vi "Data Channel Page.vi"(8 "error in (no error)":errorcluster, 11 "Node Ptr":T2 format="%.0x") -> (0 "error out":errorcluster)   [LabVIEW 2021, in "DSF System Explorer.lvlib"]
uses:
  DSF System Explorer.lvlib
  <vilib>/NI VeriStand/Custom Device API/Custom Device Item Ref.ctl
  Includes/DSF Core.lvlibp/Classes/Component User Interface/UI Type.ctl
  <vilib>/NI VeriStand/Custom Device API/Custom Device API.lvlib
  Shared/DSF Shared.lvlib
  Includes/DSF Core.lvlibp/Classes/Component User Interface/Component User Interfaces.lvclass
  Includes/DSF Core.lvlibp/Classes/User Interface/User Interface.lvclass
panel:
  in  "Tab Control":enum32{"Settings"}(tab)
  in  "Default Value":dbl
  in  "Units":string
  out "Direction":enum16{"Tx", "Rx"}(ring)
  in  "Engine Data Type":T1(ring)
  in  "String Data Type":T1(ring)
  in  "String Offset":u64 format="%d bytes"
  in  "Header":cluster{"Section Name":string}={"Section Name"="Data Channel"}
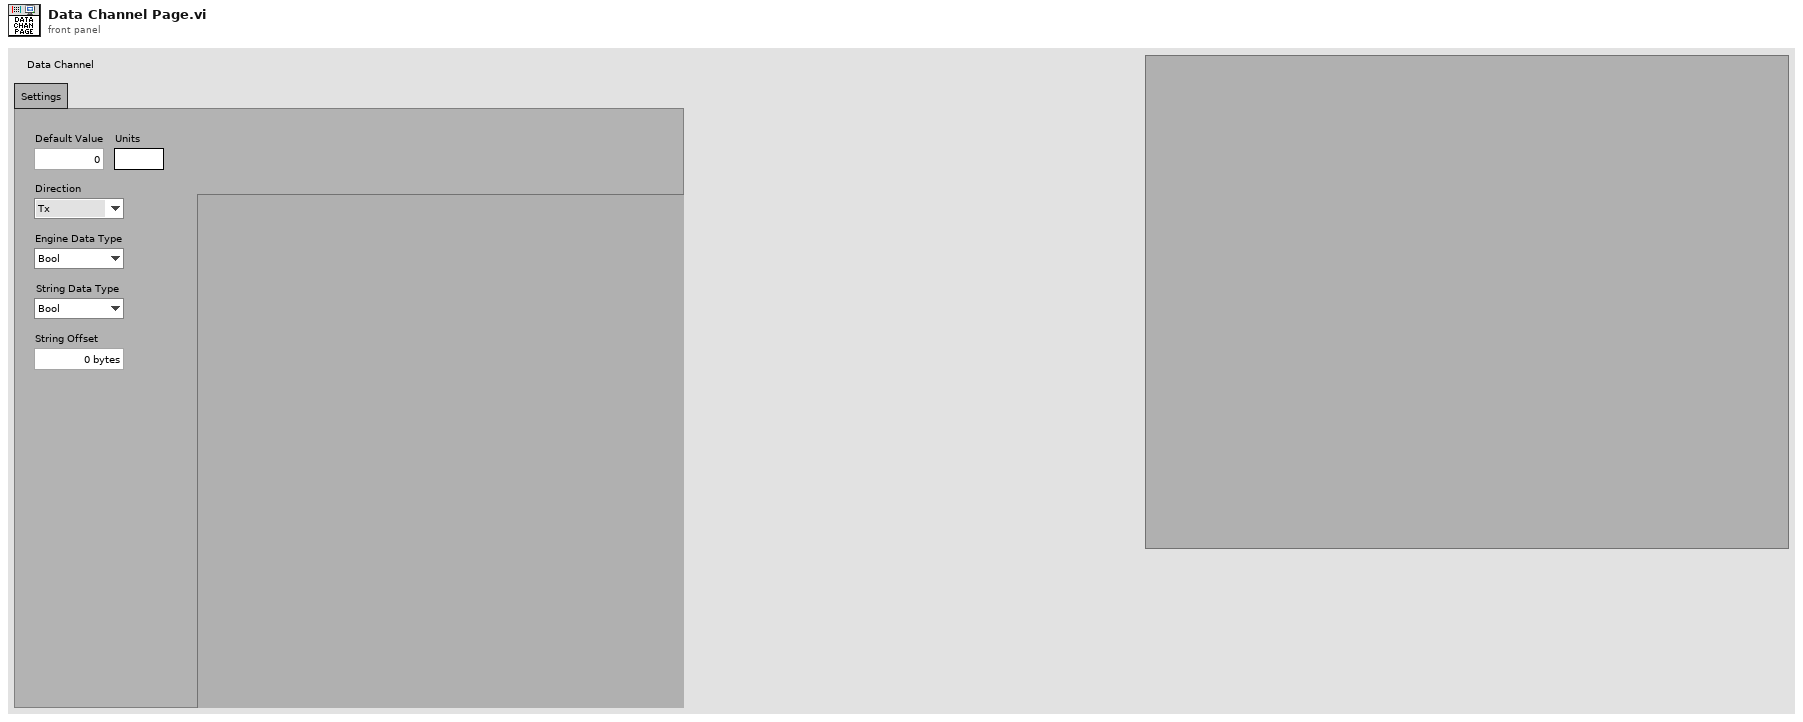
[diagram p1: front panel]
types:
  T1 = enum8{"Bool", "SGL", "DBL", "I8", "I16", "I32", "I64", "U8", "U16", "U32", "U64"}
  T2 = typedef "Custom Device API.lvlib/Custom Device Item Ref.ctl" = u64
  T3 = typedef "DSF Core.lvlibp/Component User Interfaces.lvclass/UI Type.ctl" = enum16{"Plugin", "Thread", "Rx Group", "Tx Group", "Rx Transfer", "Tx Transfer", "Rx Channel", "Tx Channel"}
  T4 = typedef "DSF Core.lvlibp/Channel Configuration.lvclass/Core Channel Configuration.ctl" = cluster{"name":string, "units":string, "engine data type":T5, "string data type":T5, "string offset":u64}
  T5 = typedef "DSF Core.lvlibp/DSF Data Type.ctl" = enum8{"Bool", "SGL", "DBL", "I8", "I16", "I32", "I64", "U8", "U16", "U32", "U64"}
  T6 = typedef "Custom Device API.lvlib/Custom Device Channel.ctl" = cluster{"Type":T7, "Units":string, "Default Value":dbl, "Faultable":bool, "Scalable":bool}
  T7 = typedef "Custom Device API.lvlib/Custom Device Channel Type.ctl" = enum16{"Input", "Output"}
  T8 = typedef "DSF Core.lvlibp/DSF Direction.ctl" = enum8{"Tx", "Rx"}
  T9 = typedef "DSF Core.lvlibp/User Interface Handler.lvclass/User Interface Ref.ctl" = refnum<vi>
  T10 = typedef "DSF Core.lvlibp/DSF Settings Info.ctl" = cluster{"component":string, "values":cluster{"key":string, "value":string}[]}
  T11 = typedef "Custom Device API.lvlib/Custom Device Commands.ctl" = enum16{"Default", "Item renamed", "Shutdown", "Dynamic button pressed"}
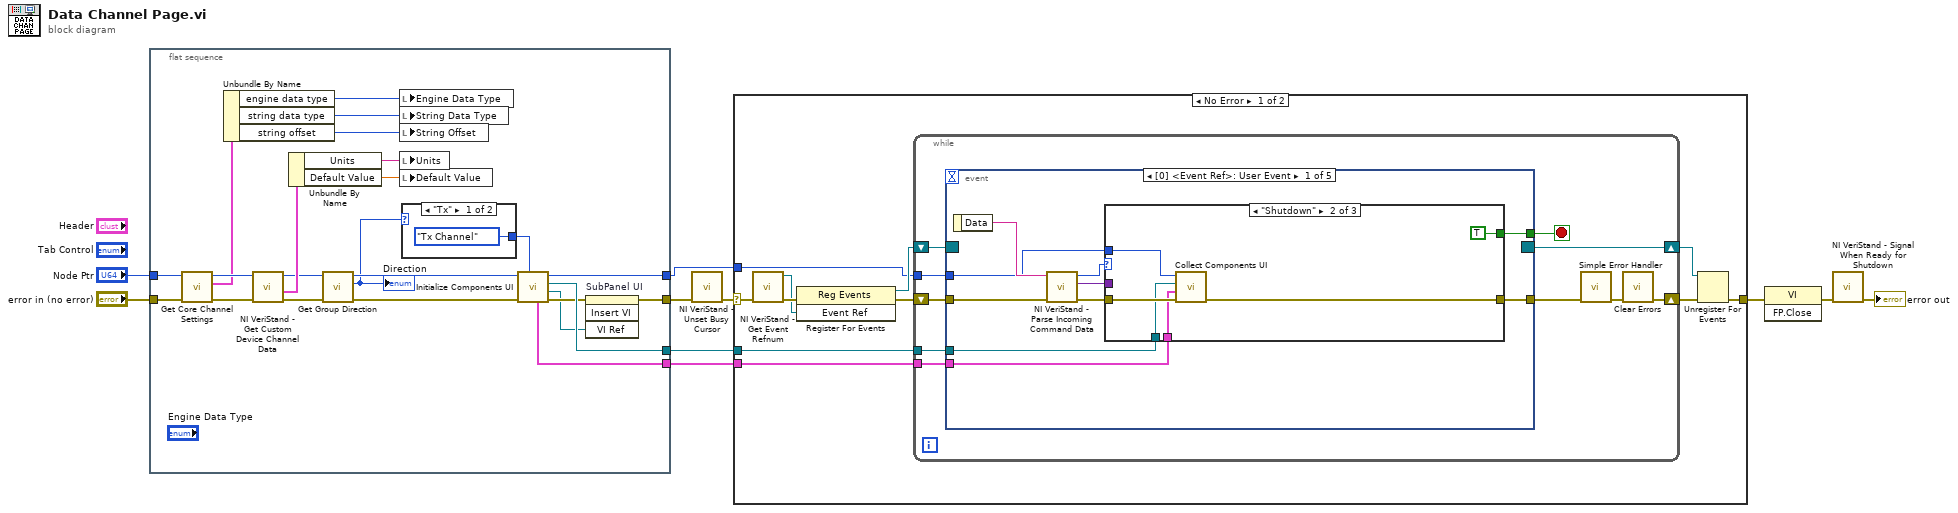
[diagram p0: block diagram]
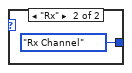
[diagram p2: hidden frame]
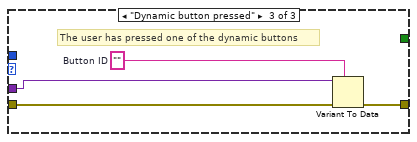
[diagram p4: hidden frame]
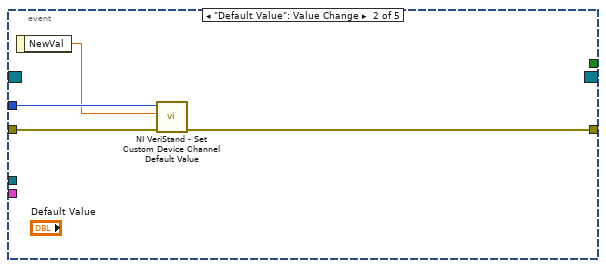
[diagram p5: hidden frame]
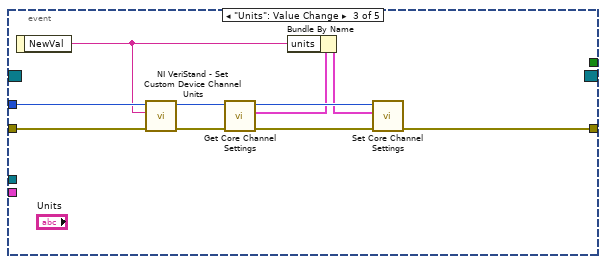
[diagram p6: hidden frame]
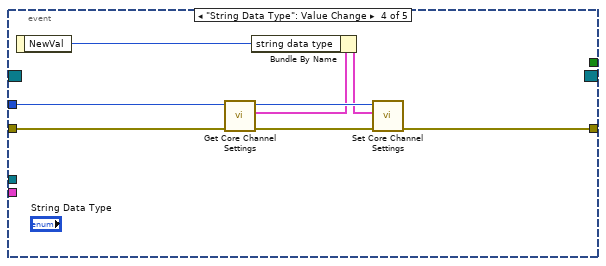
[diagram p7: hidden frame]
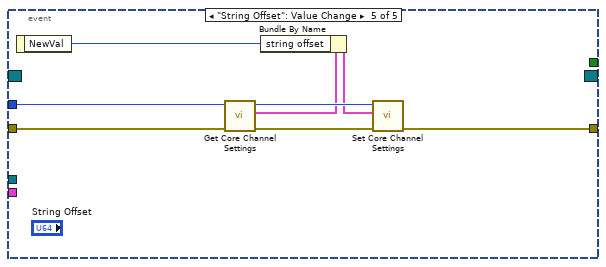
[diagram p8: hidden frame]
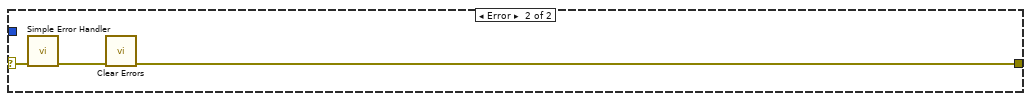
[diagram p9: hidden frame]
diagram:
  n1 = flat-sequence "Initialization code" {
    tunnel: "error in (no error)" -> [w31]
    tunnel: "Node Ptr" -> [w30]
    tunnel: [w12] -> w6
    tunnel: [w15] -> w3
    tunnel: [w16] -> w2
    tunnel: [w14] -> w1
    frame #0 {
      n2 = call "Get Core Channel Settings.vi"("error in (no error)"=w31, "Item Ref in"=w30) -> ("error out"=w29:errorcluster, "channel configuration"=w27:T4, "Item Ref out"=w28:T2)  [unwired: 7 in]
      n3 = Unbundle By Name(w27) -> ("engine data type"=w25:T5, "string data type"=w24:T5, "string offset"=w23:u64)
      n4 = call <vilib>:"NI VeriStand - Get Custom Device Channel Data.vi"("error in (no error)"=w29, "Channel Ref in"=w28) -> ("error out"=w22:errorcluster, "Channel"=w26:T6, "Channel Ref out"=w21:T2)  [unwired: 4 in, 3 out]
      n5 = Unbundle By Name(w26) -> ("Units"=w32:string, "Default Value"=w33:dbl)
      n6 = call "Get Group Direction.vi"("error in (no error)"=w22, "Item Ref in"=w21) -> ("error out"=w19:errorcluster, "direction"=w17:T8, "Item Ref out"=w18:T2)  [unwired: 6 in, 1 out]
      "Direction" <- w17
      n7 = local write "Engine Data Type"(w25) -> ()
      n8 = local write "String Data Type"(w24) -> ()
      n9 = local write "String Offset"(w23) -> ()
      n10 = local write "Units"(w32) -> ()
      n11 = local write "Default Value"(w33) -> ()
      n12 = case shown="\"Tx\"" w17 {
        tunnel: [UI_Type."Tx Channel" ("user interface type") UI_Type."Rx Channel" ("user interface type")] -> w20
        frame "Tx" {
        }
        frame "Rx" {
        }
      }
      n13 = call "Initialize Components UI.vi"("user interface type"=w20, "error in (no error)"=w19, "Item Ref in"=w18) -> ("error out"=w13:errorcluster, "active vi"=w11:T9, "User Interface Handler"=w16:refnum<class "User Interface Handler.lvclass">, "Item Ref out"=w15:T2, "component settings"=w14:T10[])  [unwired: 4 in]
      n14 = invoke on="SubPanel UI" class="SubPnl" method="Insert VI"(error in=w13, "VI Ref"=w11) -> (error out=w12:errorcluster)  [unwired: 2 in, 3 out]
    }
  }
  n15 = call <vilib>:"NI VeriStand - Unset Busy Cursor.vi"("error in (no error)"=w6) -> ("error out"=w5:errorcluster)  [unwired: 10 out]
  n16 = case shown="No Error" w5 {
    selector: w5 -> [w38 w110]
    tunnel: [w43 w108] -> w10
    tunnel: w3 -> [w39 _]
    tunnel: w2 -> [w37 _]
    tunnel: w1 -> [w36 _]
    frame No Error {
      n17 = call <vilib>:"NI VeriStand - Get Event Refnum.vi"("error in (no error)"=w38) -> ("error out"=w46:errorcluster, "Event Ref"=w42:refnum<user-event>)  [unwired: 9 out]
      n18 = register-events(error in=w46, w42) -> (reference out=w40:refnum<event-registration>, error out=w41:errorcluster)  [unwired: 1 in]
      n19 = while {
        tunnel: w39 -> [w52]
        shift-right: [w49] -> w44
        shift-left: w41 -> [w55]
        shift-right: [w56] -> w45
        shift-left: w40 -> [w54]
        tunnel: w37 -> [w48]
        tunnel: w36 -> [w47]
        stop <- w53 stop-if-true
        n20 = event shown="[0] <Event Ref>: User Event" {
          selector: w54 -> [_ _ _ _ _]
          dyn-events: [_ _ _ _ _] -> w56
          timeout: _ -> [_ _ _ _ _]
          tunnel: w55 -> [w66 w81 w91 w99 w107]
          tunnel: [w62 _ _ _ _] -> w53
          tunnel: [w61 w78 w82 w92 w100] -> w51
          tunnel: w52 -> [w60 w80 w90 w98 w106]
          tunnel: w48 -> [w58 _ _ _ _]
          tunnel: w47 -> [w57 _ _ _ _]
          event User Event {
            n21 = event-data() -> ("Data"=w65:string)  [unwired: 1 out]
            n22 = call <vilib>:"NI VeriStand - Parse Incoming Command Data.vi"("error in (no error)"=w66, "Incoming data"=w65) -> ("error out"=w64:errorcluster, "Outgoing data"=w59:variant, "Action"=w63:T11)  [unwired: 7 out]
            n23 = case shown="\"Shutdown\"" w63 {
              tunnel: w64 -> [w67 w72 w77]
              tunnel: [_ TRUE _] -> w62
              tunnel: [w67 w69 w74] -> w61
              tunnel: w60 -> [_ w71 _]
              tunnel: w59 -> [_ _ w76]
              tunnel: w58 -> [_ w70 _]
              tunnel: w57 -> [_ w68 _]
              frame "Default", Default {
              }
              frame "Shutdown" {
                n24 = call "Collect Components UI.vi"("error in (no error)"=w72, "current component settings"=w68, "User Interface Handler"=w70, "Item Ref in"=w71) -> ("error out"=w69:errorcluster)  [unwired: 6 in, 1 out]
              }
              frame "Dynamic button pressed" {
                w75 = ""  # Button ID
                # "The user has pressed one of the dynamic buttons"
                n25 = Variant To Data(error in=w77, type=w75, Variant=w76) -> (error out=w74:errorcluster)  [unwired: 1 out]
              }
            }
          }
          event "Default Value": Value Change {
            n26 = event-data() -> ("NewVal"=w79:dbl)  [unwired: 1 out]
            n27 = call <vilib>:"NI VeriStand - Set Custom Device Channel Default Value.vi"("error in (no error)"=w81, "Default Value"=w79, "Channel Ref in"=w80) -> ("error out"=w78:errorcluster)  [unwired: 7 in, 1 out]
          }
          event "Units": Value Change {
            n28 = event-data() -> ("NewVal"=w83:string)  [unwired: 1 out]
            n29 = call <vilib>:"NI VeriStand - Set Custom Device Channel Units.vi"("error in (no error)"=w91, "Units"=w83, "Channel Ref in"=w90) -> ("error out"=w89:errorcluster, "Channel Ref out"=w88:T2)  [unwired: 7 in]
            n30 = call "Get Core Channel Settings.vi"("error in (no error)"=w89, "Item Ref in"=w88) -> ("error out"=w87:errorcluster, "channel configuration"=w85:T4, "Item Ref out"=w86:T2)  [unwired: 7 in]
            n31 = Bundle By Name(cluster=w85, "units"=w83) -> (w84:T4)
            n32 = call "Set Core Channel Settings.vi"("error in (no error)"=w87, "channel configuration"=w84, "Item Ref in"=w86) -> ("error out"=w82:errorcluster)  [unwired: 7 in, 1 out]
          }
          event "String Data Type": Value Change {
            n33 = event-data() -> ("NewVal"=w93:T1)  [unwired: 1 out]
            n34 = call "Get Core Channel Settings.vi"("error in (no error)"=w99, "Item Ref in"=w98) -> ("error out"=w97:errorcluster, "channel configuration"=w95:T4, "Item Ref out"=w96:T2)  [unwired: 7 in]
            n35 = Bundle By Name(cluster=w95, "string data type"=w93) -> (w94:T4)
            n36 = call "Set Core Channel Settings.vi"("error in (no error)"=w97, "channel configuration"=w94, "Item Ref in"=w96) -> ("error out"=w92:errorcluster)  [unwired: 7 in, 1 out]
          }
          event "String Offset": Value Change {
            n37 = event-data() -> ("NewVal"=w101:u64)  [unwired: 1 out]
            n38 = call "Get Core Channel Settings.vi"("error in (no error)"=w107, "Item Ref in"=w106) -> ("error out"=w105:errorcluster, "channel configuration"=w103:T4, "Item Ref out"=w104:T2)  [unwired: 7 in]
            n39 = Bundle By Name(cluster=w103, "string offset"=w101) -> (w102:T4)
            n40 = call "Set Core Channel Settings.vi"("error in (no error)"=w105, "channel configuration"=w102, "Item Ref in"=w104) -> ("error out"=w100:errorcluster)  [unwired: 7 in, 1 out]
          }
        }
        n41 = call <vilib>:"Simple Error Handler.vi"("error in (no error)"=w51) -> ("error out"=w50:errorcluster)  [unwired: 1 in, 7 out]
        n42 = call <vilib>:"Clear Errors.vi"("error in (no error)"=w50) -> ("error out"=w49:errorcluster)  [unwired: 1 in, 5 out]
      }
      n43 = Unregister For Events(event registration refnum=w45, error in=w44) -> (error out=w43:errorcluster)
    }
    frame Error {
      n44 = call <vilib>:"Simple Error Handler.vi"("error in (no error)"=w110) -> ("error out"=w109:errorcluster)  [unwired: 1 in, 7 out]
      n45 = call <vilib>:"Clear Errors.vi"("error in (no error)"=w109) -> ("error out"=w108:errorcluster)  [unwired: 1 in, 5 out]
    }
  }
  n46 = invoke class="VI" method="FP.Close"(error in=w10) -> (error out=w9:errorcluster)  [unwired: 2 in, 2 out]
  n47 = call <vilib>:"NI VeriStand - Signal When Ready for Shutdown.vi"("error in (no error)"=w9) -> ("error out"=→"error out":errorcluster)  [unwired: 10 out]
